vi "WSVCAP SHL Host LL I2C Convert Bit Array to Channel Bytes.vi"(0 "Bit Array":u64[](array[numeric]) format="%.0x") -> (4 "C1:1-18 Read Data [SKT Ordered]":u8[][](array[numeric]) format="%.0x", 6 "C2:1-18 Read Data [SKT Ordered]":u8[][](array[numeric]) format="%.0x", 8 "C3:1-18 Read Data [SKT Ordered]":u8[][](array[numeric]) format="%.0x")   [LabVIEW 2012]
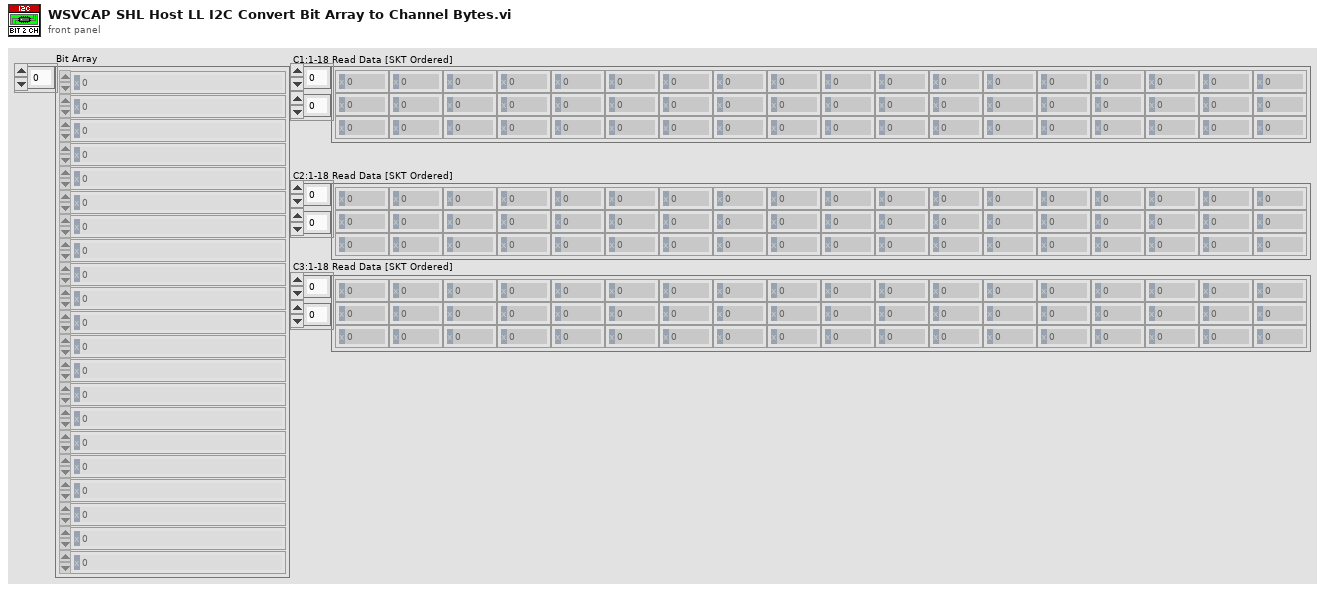
[diagram p1: front panel]
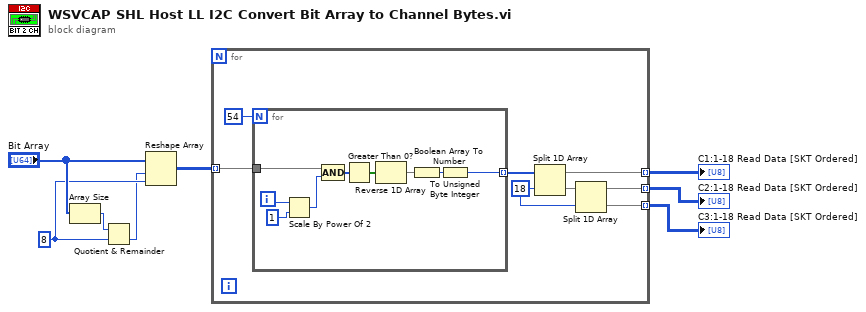
[diagram p0: block diagram]
diagram:
  w5 = 8 ("Read Data In")
  n1 = Array Size(array="Bit Array") -> (size(s)=w7:i32)
  n2 = Quotient & Remainder(x=w7, y=w5) -> (floor(x/y)=w4:i32)  [unwired: 1 out]
  n3 = Reshape Array("Bit Array", w4, w5) -> (w6:u64[][])
  n4 = for {
    tunnel: w6 -> [w16] mode=indexing
    tunnel: [w13] -> w3 mode=indexing
    tunnel: [w10] -> w2 mode=indexing
    tunnel: [w9] -> w1 mode=indexing
    w11 = 18 ("index")
    n5 = for {
      N: 54 -> [_]
      tunnel: w16 -> [w24]
      tunnel: [w20] -> w14 mode=indexing
      i -> [w19]
      n6 = Scale By Power Of 2(n=w19, x=u64 1) -> (x*2^n=w23:u64)
      n7 = Compound Arithmetic op=AND(w24, w23) -> (w22:u64[])
      n8 = Greater Than 0?(x=w22) -> (x > 0?=w18:bool[])
      n9 = Reverse 1D Array(array=w18) -> (reversed array=w17:bool[])
      n10 = Boolean Array To Number(Boolean array=w17) -> (number=w21:u32)
      n11 = To Unsigned Byte Integer(number=w21) -> (unsigned 8bit integer=w20:u8)
    }
    n12 = Split 1D Array(array=w14, index=w11) -> (first subarray=w13:u8[], second subarray=w12:u8[])
    n13 = Split 1D Array(array=w12, index=w11) -> (first subarray=w10:u8[], second subarray=w9:u8[])
  }
  "C1:1-18 Read Data [SKT Ordered]" <- w3
  "C2:1-18 Read Data [SKT Ordered]" <- w2
  "C3:1-18 Read Data [SKT Ordered]" <- w1
